vi "GetImage.vi"(8 "error in (no error)":errorcluster, 10 "Buffer Number":u32, 11 "Image Acquisition in":refnum<class "HAMAMATSU_DCAMAPI.lvclass">) -> (0 "error out":errorcluster, 1 "Cluster":cluster{"processedFPS":dbl, "Buffer Number":u32}, 2 "Image Reference":u16[][](array[numeric]), 3 "Image Acquisition out":refnum<class "HAMAMATSU_DCAMAPI.lvclass">)   [LabVIEW 2020, in "HAMAMATSU_DCAMAPI.lvclass"]
uses:
  HAMAMATSU_DCAMAPI.lvclass
  HAMAMATSU_DCAMAPI.lvclass/HAMAMATSU_DCAMAPI.ctl
panel:
  out "Timestamp":dbl
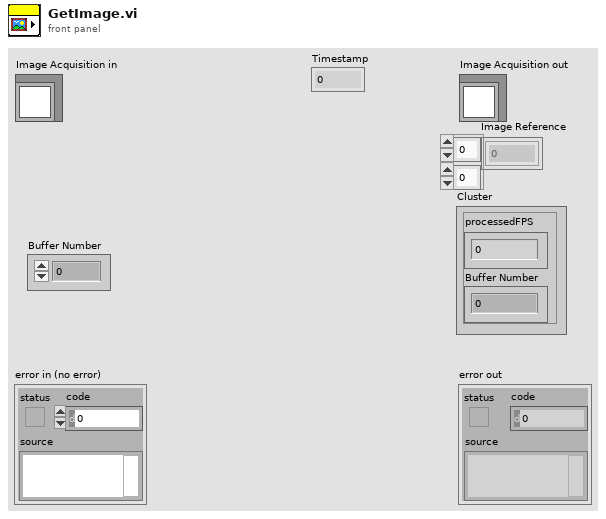
[diagram p1: front panel]
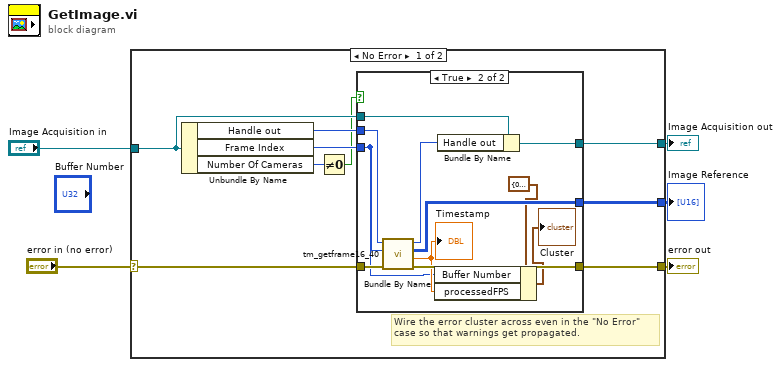
[diagram p0: block diagram]
diagram:
  n1 = case shown="No Error" "error in (no error)" {
    selector: "error in (no error)" -> [w13 w29]
    tunnel: [w12 w29] -> w5
    tunnel: [w10 w28] -> w2
    tunnel: "Image Acquisition in" -> [w11 w28]
    tunnel: [w9 _] -> w1
    frame No Error {
      # "Wire the error cluster across even in the \"No Error\"\ncase so that warnings get propagated."
      n2 = Unbundle By Name(w11) -> ("Handle out"=w14:u32, "Frame Index"=w8:i32, "Number Of Cameras"=w7:u32)
      n3 = Not Equal To 0?(x=w7) -> (x != 0?=w6:bool)
      n4 = case shown="True" w6 {
        tunnel: w14 -> [_ w27]
        tunnel: w13 -> [w15 w26]
        tunnel: [w15 w25] -> w12
        tunnel: w11 -> [w16 w24]
        tunnel: [w16 w23] -> w10
        tunnel: [_ w21] -> w9
        tunnel: w8 -> [_ w17]
        frame False {
        }
        frame True {
          n5 = call <userlib>:"tm_getframe16_40.vi"("error in (no error)"=w26, "Frame Index"=w17, "Handle in"=w27) -> ("error out"=w25:errorcluster, "Timestamp"=w20:dbl, "Data"=w21:u16[][], "Handle out"=w22:u32)  [unwired: 5 in]
          "Timestamp" <- w20
          n6 = Bundle By Name(cluster=cluster{"processedFPS":dbl, "Buffer Number":u32} {"processedFPS"=0.0, "Buffer Number"=0} ("Cluster"), "Buffer Number"=w17, "processedFPS"=w20) -> (→"Cluster":cluster{"processedFPS":dbl, "Buffer Number":u32})
          n7 = Bundle By Name(cluster=w24, "Handle out"=w22) -> (w23:refnum<class "HAMAMATSU_DCAMAPI.lvclass">)
        }
      }
    }
    frame Error {
    }
  }
  "error out" <- w5
  "Image Acquisition out" <- w2
  "Image Reference" <- w1
